vi "Set Range.vi"(8 "error in (no error)":errorcluster, 9 "Input Level":dbl, 10 "Range Array":dbl[](array[numeric])) -> (0 "error out":errorcluster, 1 "Range":dbl, 2 "In Range?":bool)   [LabVIEW 2019, in "3300.lvlib" / "3300.lvclass"]
uses:
  Library/3300.lvclass
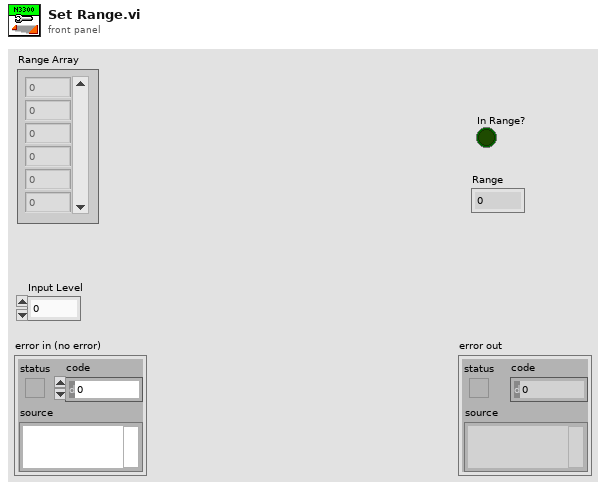
[diagram p1: front panel]
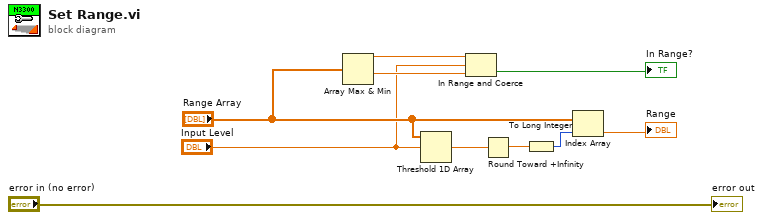
[diagram p0: block diagram]
diagram:
  n1 = Array Max & Min(array="Range Array") -> (max value=w7:dbl, min value=w6:dbl)  [unwired: 2 out]
  n2 = Threshold 1D Array(2:"Input Level", 3:"Range Array") -> (0:w9:dbl)  [unwired: 1 in]
  n3 = In Range and Coerce(upper limit=w7, x="Input Level", lower limit=w6) -> (In Range?=→"In Range?":bool)  [unwired: 1 out]
  n4 = Round Toward +Infinity(x=w9) -> (ceil(x): smallest int >= x=w4:dbl)
  n5 = To Long Integer(number=w4) -> (32bit integer=w3:i32)
  n6 = Index Array(array="Range Array", index=w3) -> (element=→"Range":dbl)
  "error out" <- "error in (no error)"
